vi "Delete.vi"(11 "Msg Output in":refnum<class "Msg Output.lvclass">) -> ()   [LabVIEW 2020, in "jettl.lvlib" / "Msg Output.lvclass"]
uses:
  Msg Output.lvclass
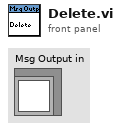
[diagram p1: front panel]
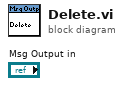
[diagram p0: block diagram]
diagram:
